vi "SAPI Select Voice SubVI.vi"(8 "error in (no error)":errorcluster, 9 "Voice Index (default voice: 0)":u16, 11 "speech object references":T1) -> (0 "error out":errorcluster, 1 "Voice Index (coerced)":u16, 3 "speech object references (out)":T1)   [LabVIEW 2021, in "SAPI.TTS.lvlib"]
doc: "Selects the SAPI voice to use for TTS."
uses:
  Users/sacha/Desktop/labview/TTS new 2012/SAPI TTS Library/SAPI.TTS.lvlib
  Users/sacha/Desktop/labview/TTS new 2012/SAPI TTS Library/Controls/Speech object references.ctl
panel:
  # "Selects the SAPI voice to use for TTS."
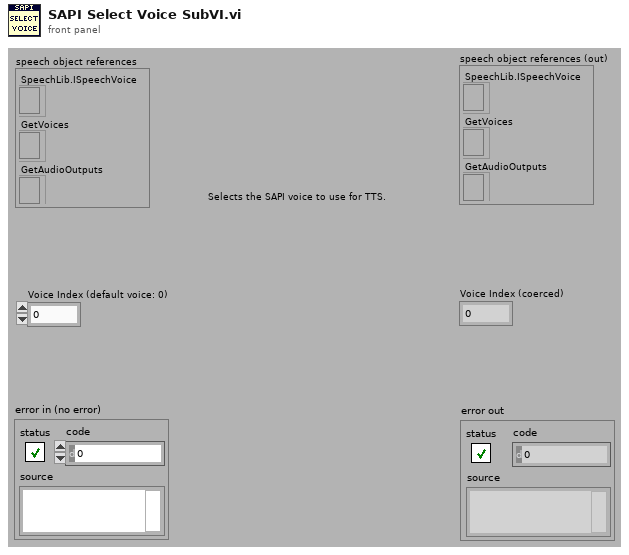
[diagram p1: front panel]
types:
  T1 = typedef "SAPI.TTS.lvlib/Speech object references.ctl" = cluster{"SpeechLib.ISpeechVoice":refnum<k7>, "GetVoices":refnum<k7>, "GetAudioOutputs":refnum<k7>}
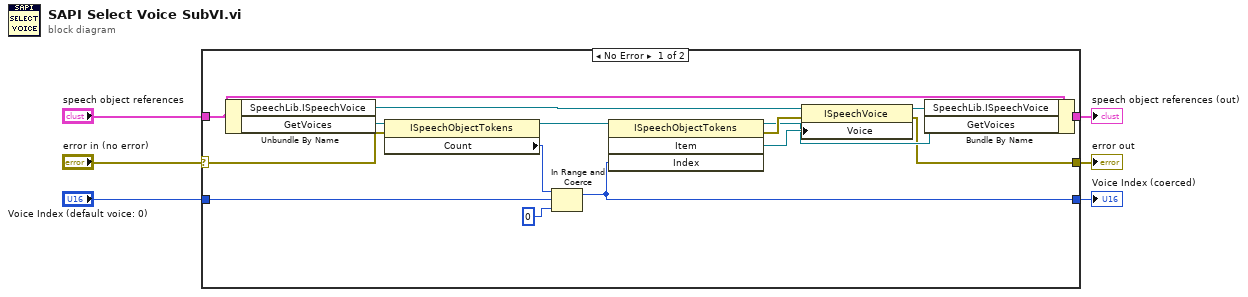
[diagram p0: block diagram]
diagram:
  n1 = case shown="No Error" "error in (no error)" {
    selector: "error in (no error)" -> [w7 w24]
    tunnel: "speech object references" -> [w18 w23]
    tunnel: [w15 w23] -> w5
    tunnel: [w14 w24] -> w4
    tunnel: "Voice Index (default voice: 0)" -> [w9 w22]
    tunnel: [w8 w22] -> w2
    frame No Error {
      n2 = Unbundle By Name(w18) -> ("SpeechLib.ISpeechVoice"=w21:refnum<k7>, "GetVoices"=w13:refnum<k7>)
      n3 = property class="ISpeechObjectTokens"(reference=w13, error in=w7) -> (reference out=w12:refnum<k7>, "Count"=w11:i32)  [unwired: 1 out]
      n4 = In Range and Coerce(upper limit=w11, x=w9, lower limit=0) -> (coerced(x)=w8:i32)  [unwired: 1 out]
      n5 = invoke class="ISpeechObjectTokens" method="Item"(reference=w12, "Index"=w8) -> (reference out=w16:refnum<k7>, error out=w20:errorcluster, "Item"=w19:refnum<k7>)  [unwired: 2 in, 1 out]
      n6 = property class="ISpeechVoice"(reference=w21, error in=w20, "Voice"=w19) -> (reference out=w17:refnum<k7>, error out=w14:errorcluster)
      n7 = Bundle By Name(cluster=w18, "SpeechLib.ISpeechVoice"=w17, "GetVoices"=w16) -> (w15:T1)
    }
    frame Error {
    }
  }
  "error out" <- w4
  "speech object references (out)" <- w5
  "Voice Index (coerced)" <- w2
